vi "Destroy.vi"(8 "error in (no error)":errorcluster, 11 "Laser Controller in":refnum<class "Laser Controller.lvclass">) -> (0 "error out":errorcluster, 3 "Laser Controller out":refnum<class "Laser Controller.lvclass">)   [LabVIEW 2022 SP3, in "Laser Controller.lvclass"]
uses:
  Laser Controller.lvclass
  Laser Controller.lvclass/Laser Controller.ctl
  XY Stage/Process Actor/Process Framework/Interlock Q Class/Interlock Q Class.lvclass
  XY Stage/Process Actor/Process Framework/Process State Data/Process State Data.lvclass
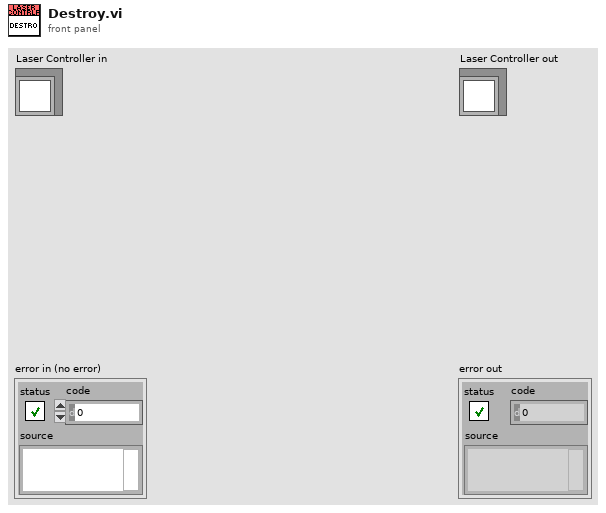
[diagram p1: front panel]
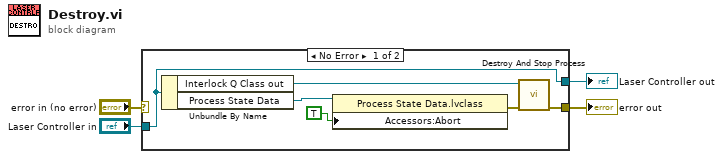
[diagram p0: block diagram]
diagram:
  n1 = case shown="No Error" "error in (no error)" {
    selector: "error in (no error)" -> [_ w12]
    tunnel: [w8 w12] -> w3
    tunnel: [w10 w11] -> w1
    tunnel: "Laser Controller in" -> [w10 w11]
    frame No Error {
      n2 = Unbundle By Name(w10) -> ("Interlock Q Class out"=w9:refnum<class "Interlock Q Class.lvclass">, "Process State Data"=w7:refnum<data-value>)
      n3 = property class="Process State Data.lvclass"(reference=w7, "Accessors:Abort"=TRUE ("Abort")) -> (error out=w5:errorcluster)  [unwired: 1 in, 1 out]
      n4 = call-dynamic "Destroy And Stop Process.vi"("error in (no error)"=w5, "Interlock Q Class in"=w9) -> ("error out"=w8:errorcluster)  [unwired: 8 in, 1 out]
    }
    frame Error {
    }
  }
  "error out" <- w3
  "Laser Controller out" <- w1
